vi "Test Load Instruments 1.vi"(11 "Test Case In":refnum<class "Test Instrument Manager.lvclass">) -> (0 "error out":errorcluster, 3 "Test Case Out":refnum<class "Test Instrument Manager.lvclass">)   [LabVIEW 2024, in "Test Instrument Manager.lvclass"]
uses:
  Test Instrument Manager.lvclass
  C:/Program Files/National Instruments/LabVIEW 2025/vi.lib/Astemes/LUnit/Test Case.lvclass
  <vilib>/Astemes/LUnit/Test Case.lvclass/Test Case.ctl
  Instrument Manager/Instrument Manager.lvclass
  <vilib>/Astemes/LUnit/Test Case.lvclass
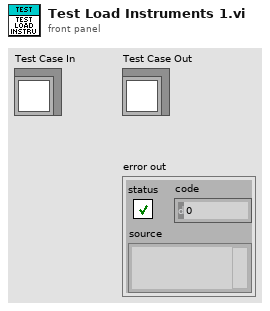
[diagram p1: front panel]
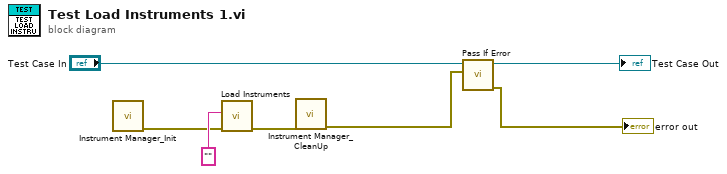
[diagram p0: block diagram]
diagram:
  n1 = call "Instrument Manager_Init.vi"() -> ("Error Out"=w4:errorcluster)  [unwired: 10 in, 1 out]
  n2 = call "Load Instruments.vi"("Error In"=w4, "Source"="") -> ("Error Out"=w3:errorcluster)  [unwired: 9 in]
  n3 = call "Instrument Manager_CleanUp.vi"("Error In"=w3) -> ("Error Out"=w2:errorcluster)  [unwired: 10 in]
  n4 = call <vilib>:"Pass If Error.vi"("Assert error"=w2, "LUnit Test Case In"="Test Case In") -> ("error out"=→"error out":errorcluster, "LUnit Test Case Out"=→"Test Case Out":refnum<class "Test Instrument Manager.lvclass">)  [unwired: 8 in]
